vi "Temp_CV.vi"() -> ()   [LabVIEW 2021]
uses:
  <vilib>/Analysis/1siggen.llb/Ramp Pattern by Samples.vi
  <vilib>/Analysis/baseanly.llb/Mean (DBL).vi
  <vilib>/Utility/file.llb/Write Delimited Spreadsheet (DBL).vi
  C:/Program Files/Metrohm Autolab/Autolab SDK 2.1/EcoChemie.Autolab.Sdk.dll
  EcoChemie.Autolab.Sdk.dll
  <vilib>/Analysis/NI_AALBase.lvlib
panel:
  out "Ramp Pattern":dbl[](array[numeric])
  in  "Stop Echem":bool
  out "Heater":bool
  out "Water Temp":dbl
  in  "Sample size":i32=56
  in  "T start":dbl=5.0 format="%0.2f"
  in  "T end":dbl=60.0 format="%0.2f"
  out "Temp LED":bool
  out "Y_array":dbl[](array[numeric])
  out "X_array":dbl[](array[numeric])
  out "y":dbl
  out "x":dbl
  in  "Signal Y sel":string(combo)="WE(1).Current"
  in  "Signal X sel":string(combo)="WE(1).Potential"
  in  "Nox file":path=path "C:/Users/YCL Lab/Documents/NOVA 2.1/Procedures/Cyclic voltammetry.nox"
  out "Rxn Temp":dbl
  out "Status":string
  out "IsMeasuring":bool
  out "jV Graph":cluster{"Values":dbl[], "Values":dbl[]}(graph)
  out "Potentiostat Connected?":bool
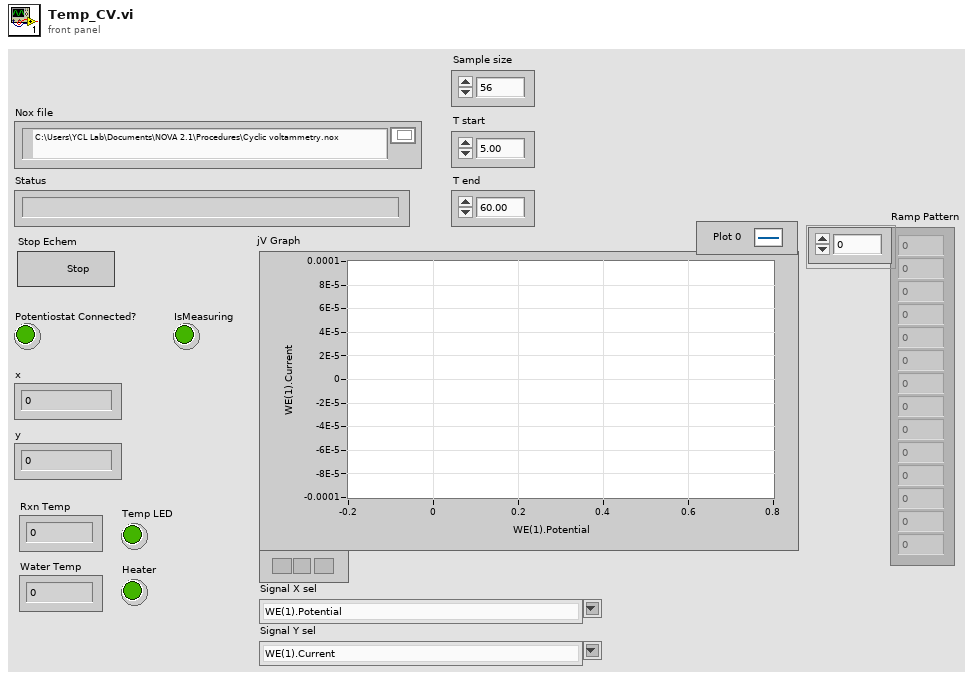
[diagram p1: front panel]
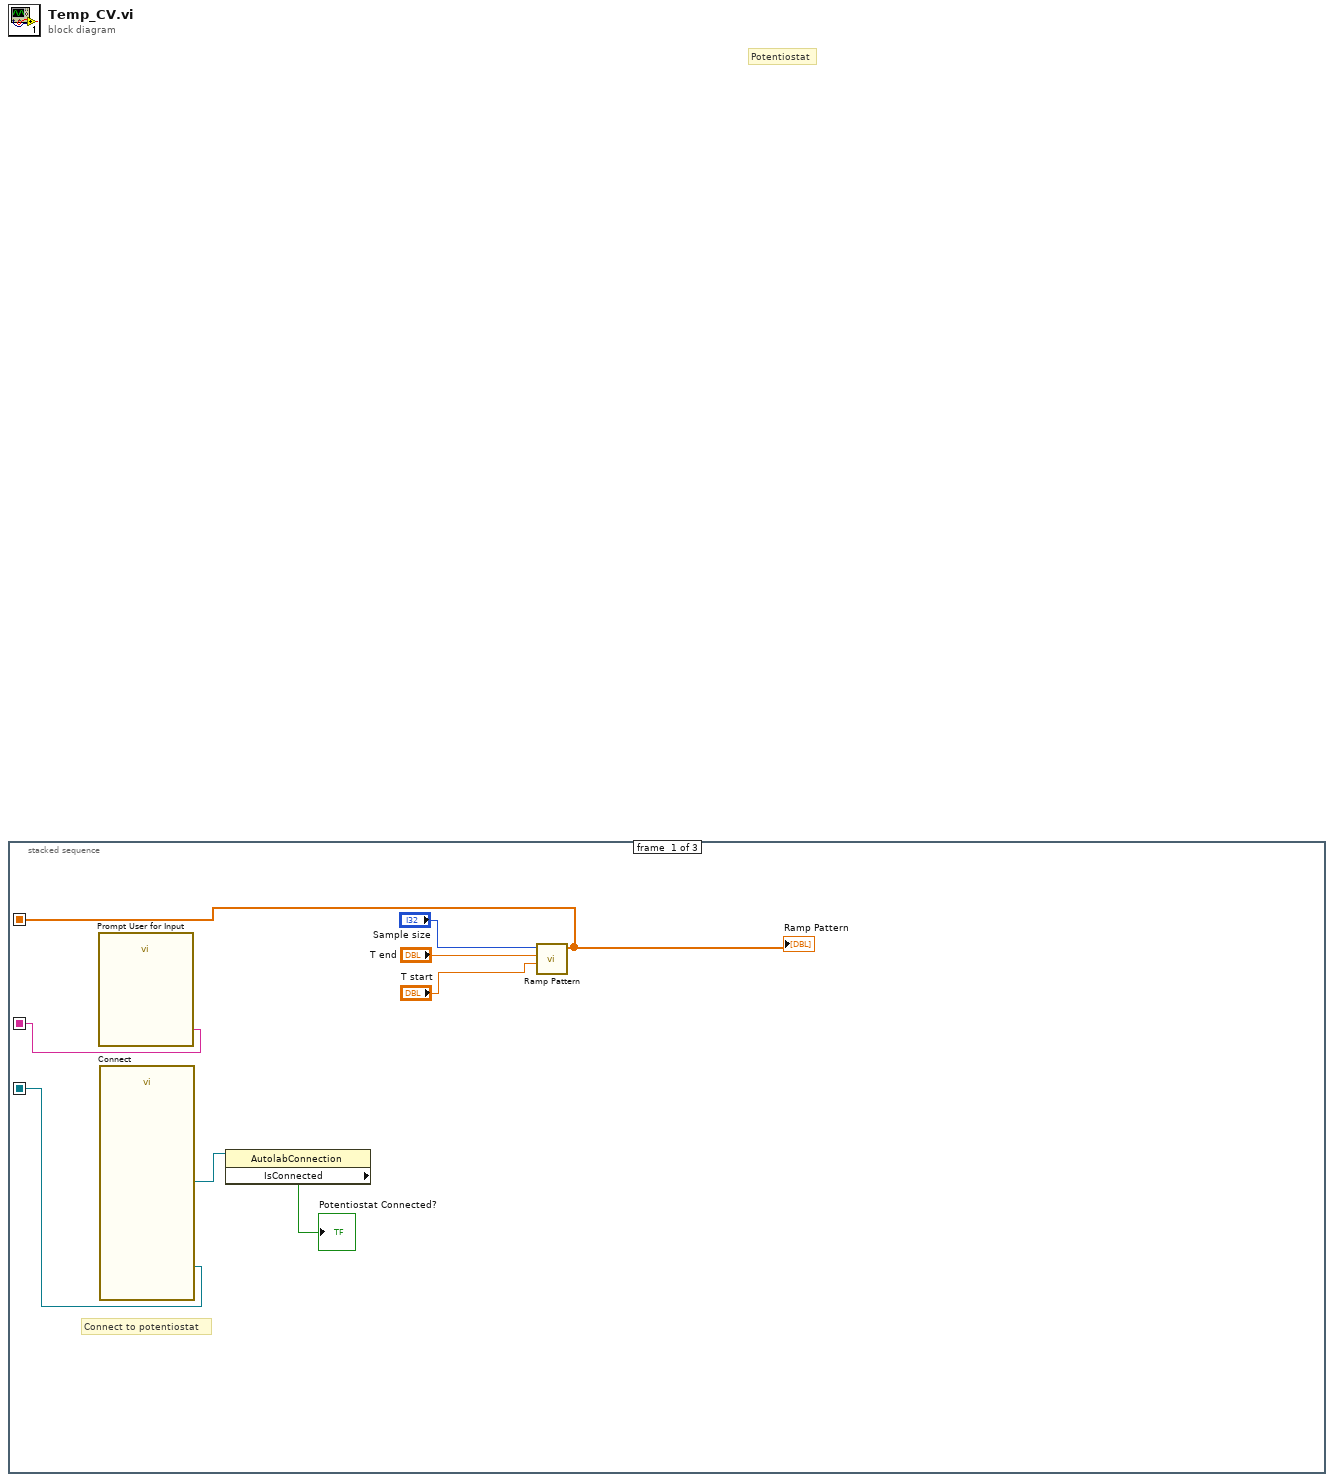
[diagram p0: block diagram]
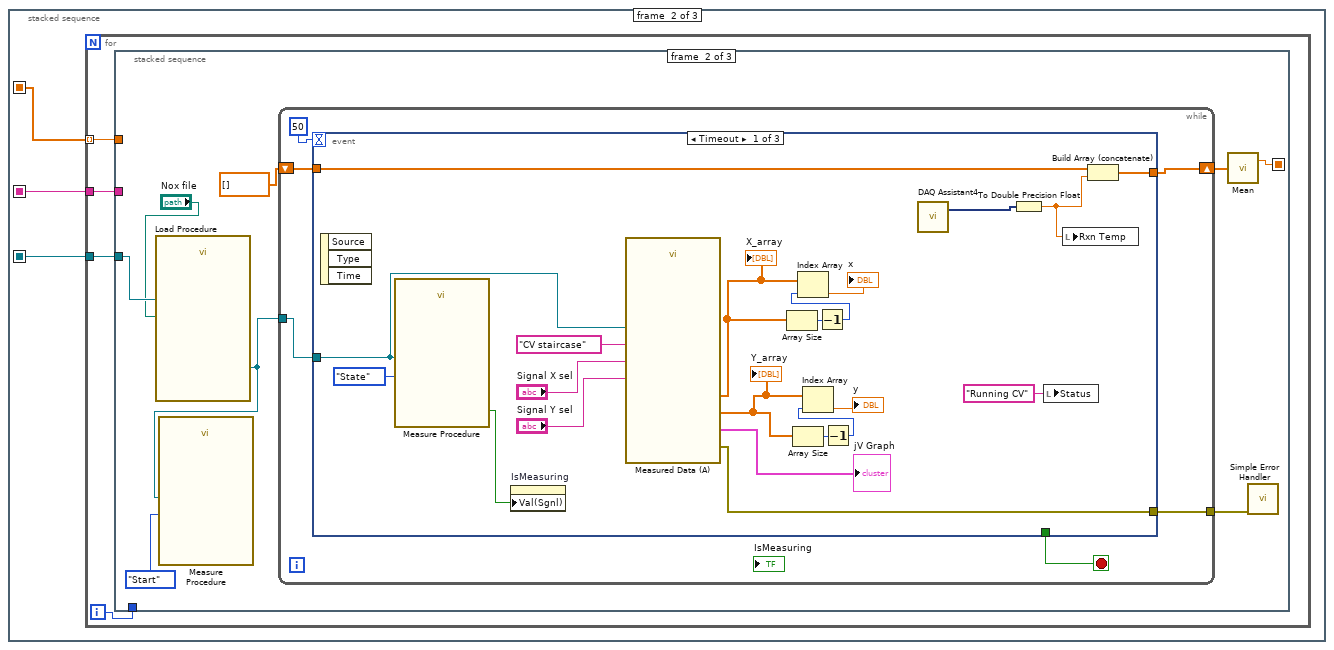
[diagram p2: hidden frame]
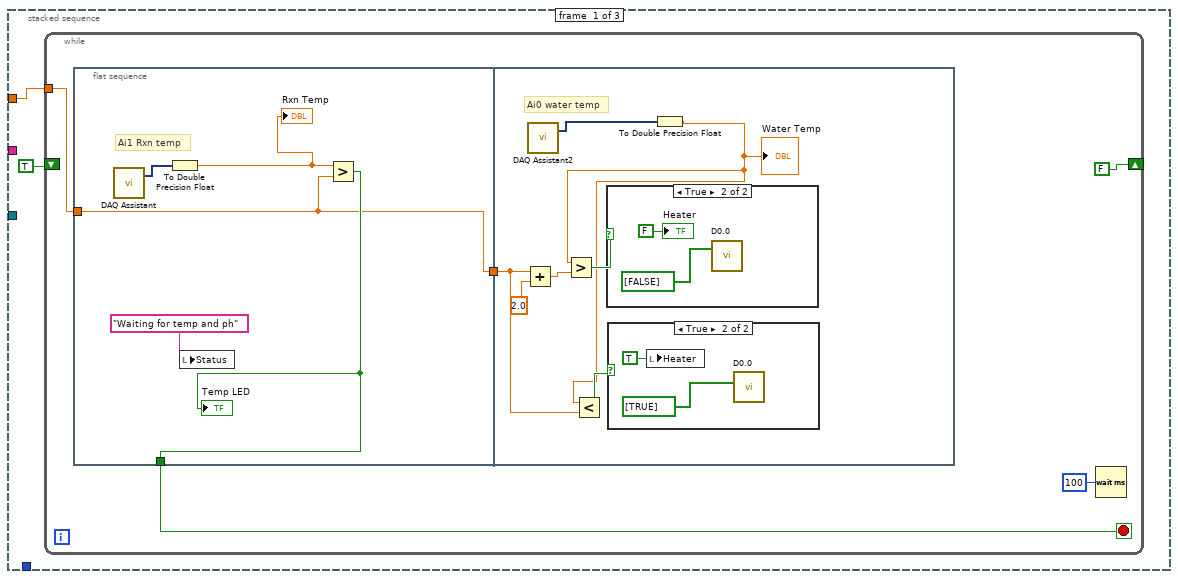
[diagram p3: hidden frame]
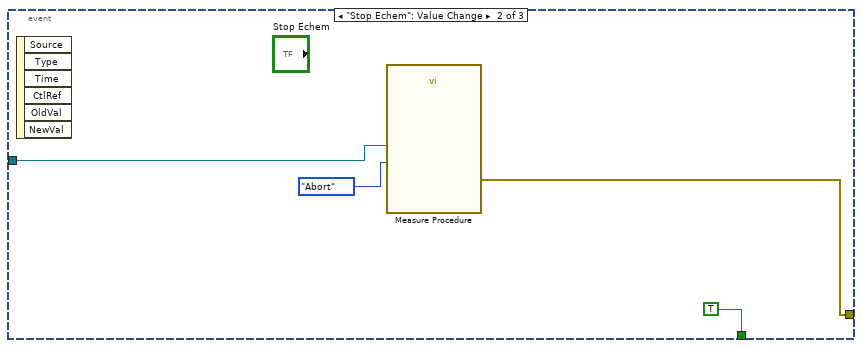
[diagram p6: hidden frame]
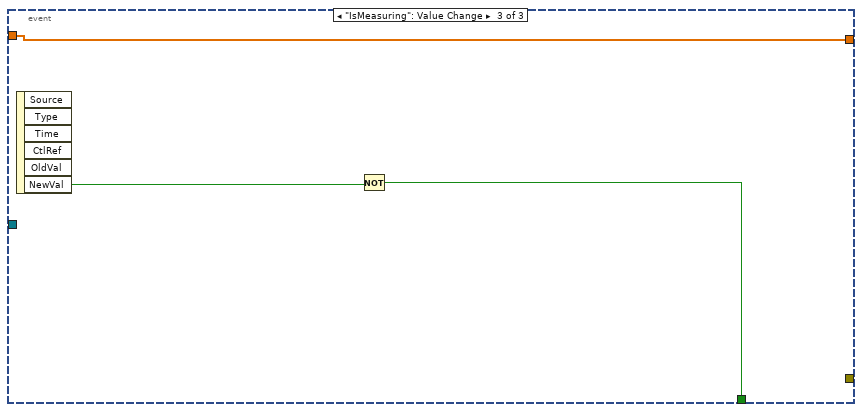
[diagram p7: hidden frame]
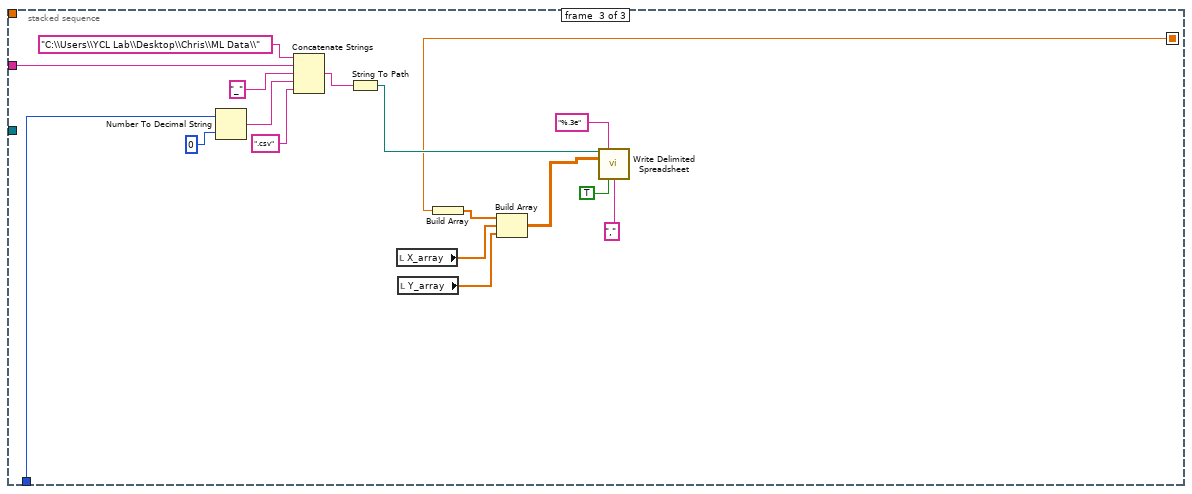
[diagram p8: hidden frame]
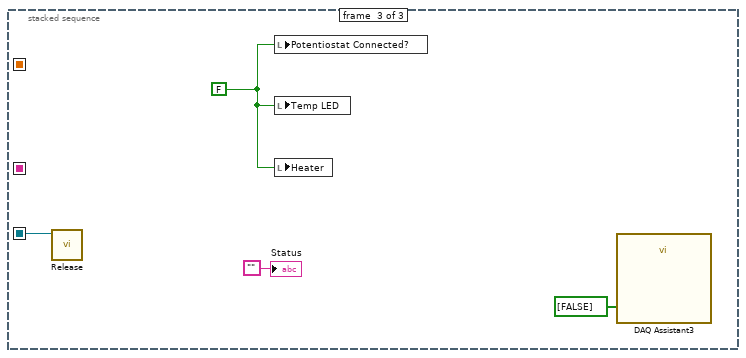
[diagram p9: hidden frame]
diagram:
  # "Potentiostat"
  n1 = stacked-sequence {
    seq-local: [w6 _ _] -> [_ w11 w101]
    seq-local: [w5 _ _] -> [_ w10 _]
    seq-local: [w1 _ _] -> [_ w9 _]
    frame #0 {
      # "Connect to potentiostat"
      n2 = call "Prompt User for Input"() -> ("File name"=w5:string)  [unwired: 17 in, 2 out]
      n3 = call "Connect.vi"() -> ("AutolabConnection"=w8:refnum<k24>, "instrument"=w6:refnum<k24>)  [unwired: 8 in, 6 out]
      n4 = property class="AutolabConnection"(reference=w8) -> ("IsConnected"=→"Potentiostat Connected?":bool)  [unwired: 1 in, 2 out]
      n5 = call-poly <vilib>:"Ramp Pattern.vi"("start"="T start", "end"="T end", "samples"="Sample size") -> ("Ramp Pattern"=w1:dbl[])  [unwired: 7 in, 1 out]
      "Ramp Pattern" <- w1
    }
    frame #1 {
      n6 = for {
        tunnel: w9 -> [w14] mode=indexing
        tunnel: w11 -> [w15]
        tunnel: w10 -> [w12]
        i -> [w13]
        n7 = stacked-sequence {
          seq-local: [_ w40 _] -> [_ _ w82]
          tunnel: w15 -> [_ w44 _]
          tunnel: w14 -> [w17 _ _]
          tunnel: w13 -> [_ _ w93]
          tunnel: w12 -> [_ _ w86]
          frame #0 {
            n8 = while {
              tunnel: w17 -> [w21]
              shift-right: [FALSE] -> _
              shift-left: TRUE -> [_]
              stop <- w19 stop-if-true
              n9 = flat-sequence {
                tunnel: [w26] -> w19
                tunnel: w21 -> [w24]
                tunnel: [w24] -> w18
                tunnel: w18 -> [w29]
                frame #0 {
                  # "Ai1 Rxn temp"
                  n10 = call "DAQ Assistant"() -> ("data"=w23:dynamicdata)  [unwired: 17 in, 2 out]
                  n11 = To Double Precision Float(number=w23) -> (double precision float=w25:dbl)
                  "Rxn Temp" <- w25
                  n12 = local write "Status"("Waiting for temp and ph" ("Status")) -> ()
                  n13 = Greater?(x=w25, y=w24) -> (0:w26:bool)
                  "Temp LED" <- w26
                }
                frame #1 {
                  # "Ai0 water temp"
                  n14 = Add(x=w29, y=2.0) -> (x+y=w34:dbl)
                  n15 = call "DAQ Assistant2"() -> ("data"=w28:dynamicdata)  [unwired: 17 in, 2 out]
                  n16 = To Double Precision Float(number=w28) -> (double precision float=w30:dbl)
                  "Water Temp" <- w30
                  n17 = Greater?(x=w30, y=w34) -> (0:w32:bool)
                  n18 = Less?(x=w30, y=w29) -> (x < y?=w31:bool)
                  n19 = case shown="True" w32 {
                    frame False {
                    }
                    frame True {
                      n20 = call "D0.0"("data"=bool[] [FALSE]) -> ()  [unwired: 17 in, 2 out]
                      "Heater" <- FALSE ("Heater")
                    }
                  }
                  n21 = case shown="True" w31 {
                    frame False {
                    }
                    frame True {
                      n22 = local write "Heater"(TRUE ("Heater")) -> ()
                      n23 = call "D0.0"("data"=bool[] [TRUE]) -> ()  [unwired: 17 in, 2 out]
                    }
                  }
                }
              }
              n24 = Wait (ms)(milliseconds to wait=u32 100) -> ()  [unwired: 1 out]
            }
          }
          frame #1 {
            n25 = call "Load Procedure.vi"("Procedure"="Nox file", "Instrument"=w44) -> ("LoadProcedure"=w46:refnum<k24>)  [unwired: 6 in, 3 out]
            n26 = call "Measure Procedure.vi"("Request for procedure"=enum16{"State", "Save", "Abort", "Start"}."Start", "LoadProcedure"=w46) -> ()  [unwired: 8 in, 2 out]
            n27 = while {
              tunnel: w46 -> [w50]
              tunnel: [w49] -> w42
              shift-right: [w48] -> w41
              shift-left: dbl[] [] -> [w47]
              stop <- w51 stop-if-true
              n28 = event shown="[0] Timeout" {
                selector: _ -> [_ _ _]
                dyn-events: _ -> [_ _ _]
                timeout: 50 -> [_ _ _]
                tunnel: [_ TRUE w79] -> w51
                tunnel: w50 -> [w69 w77 _]
                tunnel: [w57 w74 _] -> w49
                tunnel: [w56 _ w78] -> w48
                tunnel: w47 -> [w55 _ w78]
                event Timeout {
                  n29 = event-data() -> ()  [unwired: 1 in, 3 out]
                  n30 = call "Measure Procedure.vi"("Request for procedure"=enum16{"State", "Save", "Abort", "Start"}."State", "LoadProcedure"=w69) -> ("IsMeasuring"=w72:bool)  [unwired: 8 in, 1 out]
                  n31 = property on="IsMeasuring" class="Bool (strict)"("Val(Sgnl)"=w72) -> ()  [unwired: 2 in, 2 out]
                  n32 = call "Measured Data (A).vi"("LoadProcedure"=w69, "ProcedureCommandList"="CV staircase", "Signal X sel"="Signal X sel", "Signal Y sel"="Signal Y sel") -> ("Value Y"=w58:dbl[], "Value X"=w64:dbl[], "XY Graph"=→"jV Graph":cluster{"Values":dbl[], "Values":dbl[]}, "error out"=w57:errorcluster)  [unwired: 5 in, 3 out]
                  "X_array" <- w64
                  "Y_array" <- w58
                  n33 = Array Size(array=w64) -> (size(s)=w65:i32)
                  n34 = Array Size(array=w58) -> (size(s)=w61:i32)
                  n35 = Decrement(x=w65) -> (x-1=w63:i32)
                  n36 = Index Array(array=w64, index=w63) -> (element=→"x":dbl)
                  n37 = Decrement(x=w61) -> (x-1=w60:i32)
                  n38 = Index Array(array=w58, index=w60) -> (element=→"y":dbl)
                  n39 = call "DAQ Assistant4"() -> ("data"=w53:dynamicdata)  [unwired: 17 in, 2 out]
                  n40 = To Double Precision Float(number=w53) -> (double precision float=w54:dbl)
                  n41 = local write "Status"("Running CV" ("Status")) -> ()
                  n42 = local write "Rxn Temp"(w54) -> ()
                  n43 = Build Array (concatenate)(w55, w54) -> (w56:dbl[])
                }
                event "Stop Echem": Value Change {
                  n44 = event-data() -> ()  [unwired: 1 in, 6 out]
                  n45 = call "Measure Procedure.vi"("Request for procedure"=enum16{"State", "Save", "Abort", "Start"}."Abort", "LoadProcedure"=w77) -> ("error out"=w74:errorcluster)  [unwired: 8 in, 1 out]
                }
                event "IsMeasuring": Value Change {
                  n46 = event-data() -> ("NewVal"=w80:bool)  [unwired: 1 in, 5 out]
                  n47 = Not(x=w80) -> (.not. x?=w79:bool)
                }
              }
            }
            n48 = call-poly <vilib>:"Mean.vi"("X"=w41) -> ("mean"=w40:dbl)  [unwired: 1 out]
            n49 = call <vilib>:"Simple Error Handler.vi"("error in (no error)"=w42) -> ()  [unwired: 4 in, 5 out]
          }
          frame #2 {
            n50 = Number To Decimal String(number=w93, width (-)=i16 0) -> (decimal integer string=w84:string)
            n51 = Concatenate Strings("C:\\Users\\YCL Lab\\Desktop\\Chris\\ML Data\\", w86, "_" ("string"), w84, ".csv" ("string")) -> (w91:string)
            n52 = String To Path(string=w91) -> (path=w90:path)
            n53 = local read "X_array"() -> (w97:dbl[])
            n54 = local read "Y_array"() -> (w96:dbl[])
            n55 = Build Array(w82) -> (w81:dbl[])
            n56 = Build Array(w81, w97, w96) -> (w95:dbl[][])
            n57 = call-poly <vilib>:"Write Delimited Spreadsheet.vi"("file path (dialog if empty)"=w90, "format (%.3f)"="%.3e", "2D data"=w95, "transpose? (no:F)"=TRUE, "delimiter (\\t)"="," ("delimiter (\\t)")) -> ()  [unwired: 9 in, 2 out]
          }
        }
      }
    }
    frame #2 {
      w99 = FALSE ("pH LED")
      n58 = call "Release.vi"("Instrument"=w101) -> ()  [unwired: 10 in, 1 out]
      n59 = local write "Potentiostat Connected?"(w99) -> ()
      n60 = local write "Temp LED"(w99) -> ()
      n61 = local write "Heater"(w99) -> ()
      n62 = call "DAQ Assistant3"("data"=bool[] [FALSE]) -> ()  [unwired: 17 in, 2 out]
      "Status" <- ""
    }
  }
